vi "DigitalOutput Interface.vi"(8 "Eventstring":string, 9 "Pulse duration (-1 for cont.)":i32, 10 "On/off":bool=TRUE, 11 "Port index":i32) -> (1 "OutputRequest":T1)   [LabVIEW 2015]
doc: "Makes OutputRequest objects compatible with the DigitalOutput output driver.\n\n\"Port index\": Port number as indexed by the DigitalOutput driver (refer to port table)\n\"On/Off\": How to drive the line (default = true = on)\n\"Pulse ms\": Pulse duration in ms, or -1 for continuous\n\"Eventstring\": String to send w/ timestamp, or empty/unwired for no timestamp"
uses:
  Typedefs/OutputRequest.ctl
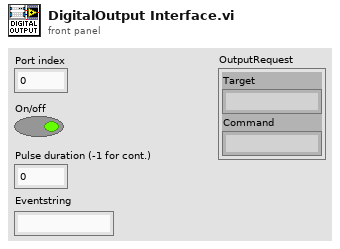
[diagram p1: front panel]
types:
  T1 = typedef "OutputRequest.ctl" = cluster{"Target":string, "Command":string}
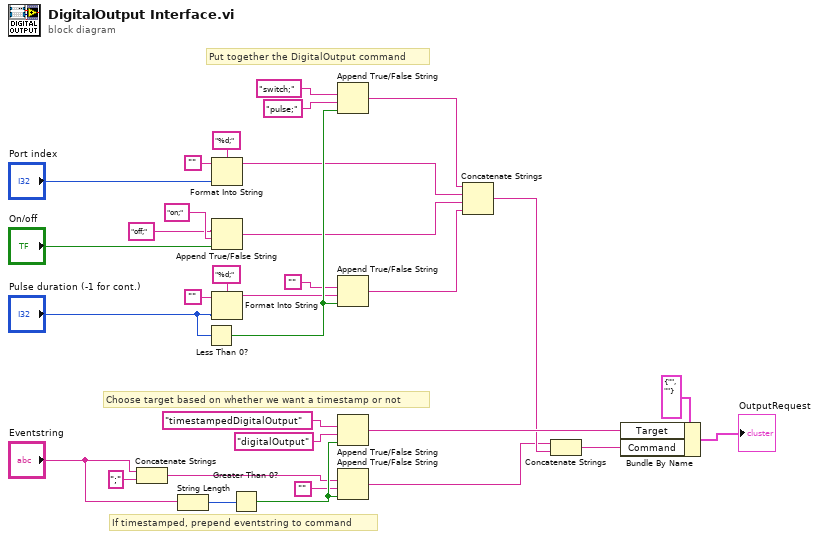
[diagram p0: block diagram]
diagram:
  # "If timestamped, prepend eventstring to command"
  # "Choose target based on whether we want a timestamp or not"
  # "Put together the DigitalOutput command"
  n1 = Concatenate Strings("Eventstring", ";" ("string")) -> (w7:string)
  n2 = String Length(string="Eventstring") -> (length=w14:i32)
  n3 = Less Than 0?(x="Pulse duration (-1 for cont.)") -> (x < 0?=w29:bool)
  n4 = Format Into String(format string="%d;", initial string="", "Port index") -> (resulting string=w18:string)  [unwired: 1 in, 1 out]
  n5 = Append True/False String(1:"On/off", 2:"on;" ("true string"), 3:"off;" ("false string")) -> (0:w17:string)  [unwired: 1 in]
  n6 = Format Into String(format string="%d;", initial string="", "Pulse duration (-1 for cont.)") -> (resulting string=w23:string)  [unwired: 1 in, 1 out]
  n7 = Greater Than 0?(x=w14) -> (x > 0?=w8:bool)
  n8 = Append True/False String(1:w29, 2:"pulse;" ("false string"), 3:"switch;" ("true string")) -> (0:w19:string)  [unwired: 1 in]
  n9 = Append True/False String(1:w29, 2:w23, 3:"") -> (0:w15:string)  [unwired: 1 in]
  n10 = Append True/False String(1:w8, 2:"digitalOutput" ("false string"), 3:"timestampedDigitalOutput" ("true string")) -> (0:w11:string)  [unwired: 1 in]
  n11 = Append True/False String(1:w8, 2:"", 3:w7) -> (0:w3:string)  [unwired: 1 in]
  n12 = Concatenate Strings(w19, w18, w17, w15) -> (w4:string)
  n13 = Concatenate Strings(w3, w4) -> (w5:string)
  n14 = Bundle By Name(cluster=T1 {"Target"="", "Command"=""} ("OutputRequest"), "Target"=w11, "Command"=w5) -> (→"OutputRequest":T1)
